vi "IP Reporter PythonCode Folder.vi"() -> ()   [LabVIEW 2017]
panel:
  out "PythonCode":path
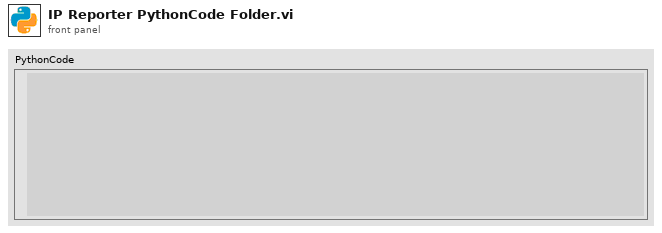
[diagram p1: front panel]
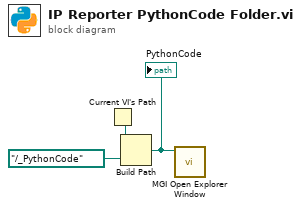
[diagram p0: block diagram]
diagram:
  n1 = Current VI's Path() -> (path=w3:path)
  n2 = Build Path(base path=w3, name or relative path=path "../_PythonCode") -> (appended path=w1:path)
  "PythonCode" <- w1
  n3 = call <userlib>:"MGI Open Explorer Window.vi"("Directory or File"=w1) -> ()  [unwired: 10 in, 1 out]
